vi "Window Maker.vi"(11 "Simple Windows":i32[][](array[numeric])) -> (3 "Plot Bounds":T1[](array[typedef]) {"Plot Bounds (%)"."Bottom (%)" format="%.2f"; "Plot Bounds (%)"."Top (%)" format="%.2f"; "Plot Bounds (%)"."Right (%)" format="%.2f"; "Plot Bounds (%)"."Left (%)" format="%.2f"})   [LabVIEW 2021, in "MultiStokePlot.lvlib" / "MultiPlotPanel.lvclass"]
uses:
  Classes/MultiPlotPanel/MultiPlotPanel.lvclass
  Window Position and plot number.ctl
  Window Position.ctl
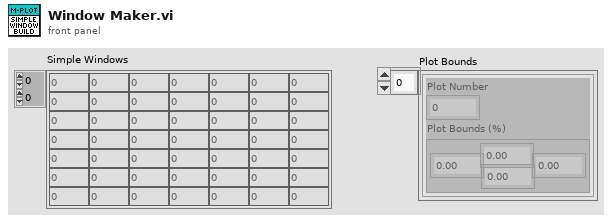
[diagram p1: front panel]
types:
  T1 = typedef "MultiStokePlot.lvlib/MultiPlotPanel.lvclass/Window Position and plot number.ctl" = cluster{"Plot Number":i32, "Plot Bounds (%)":T2}
  T2 = typedef "MultiStokePlot.lvlib/MultiPlotPanel.lvclass/Window Position.ctl" = cluster{"Left (%)":dbl, "Top (%)":dbl, "Right (%)":dbl, "Bottom (%)":dbl}
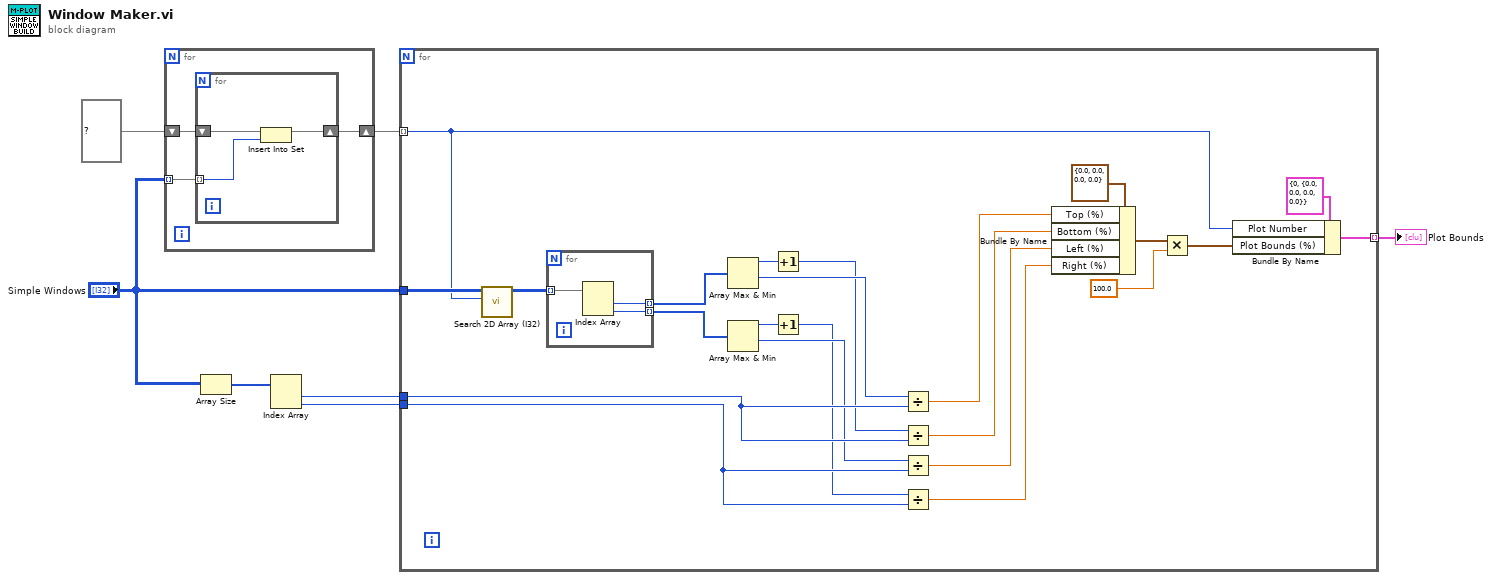
[diagram p0: block diagram]
diagram:
  n1 = for {
    tunnel: "Simple Windows" -> [w10] mode=indexing
    shift-right: [w8] -> w6
    shift-left: set{i32} {} ("set in") -> [w9]
    n2 = for {
      tunnel: w10 -> [w13] mode=indexing
      shift-right: [w11] -> w8
      shift-left: w9 -> [w12]
      n3 = Insert Into Set(10:w13, 11:w12) -> (3:w11:set{i32})  [unwired: 1 out]
    }
  }
  n4 = Array Size(array="Simple Windows") -> (size(s)=w2:i32[])
  n5 = Index Array(array=w2) -> (element #1=w4:i32, element #2=w3:i32)  [unwired: 2 in]
  n6 = for {
    tunnel: "Simple Windows" -> [w36]
    tunnel: w6 -> [w15] mode=indexing
    tunnel: w4 -> [w28]
    tunnel: w3 -> [w31]
    tunnel: [w14] -> w1 mode=indexing
    n7 = call "Search 2D Array (I32).vi"("Element"=w15, "Array"=w36) -> ("Locations"=w35:i32[][])  [unwired: 9 in]
    n8 = for {
      tunnel: w35 -> [w39] mode=indexing
      tunnel: [w38] -> w34 mode=indexing
      tunnel: [w37] -> w33 mode=indexing
      n9 = Index Array(array=w39) -> (element #1=w38:i32, element #2=w37:i32)  [unwired: 2 in]
    }
    n10 = Array Max & Min(array=w34) -> (max value=w25:i32, min value=w27:i32)  [unwired: 2 out]
    n11 = Array Max & Min(array=w33) -> (max value=w23:i32, min value=w26:i32)  [unwired: 2 out]
    n12 = Increment(x=w25) -> (x+1=w24:i32)
    n13 = Increment(x=w23) -> (x+1=w22:i32)
    n14 = Divide(x=w27, y=w28) -> (x/y=w30:dbl)
    n15 = Divide(x=w24, y=w28) -> (x/y=w21:dbl)
    n16 = Divide(x=w26, y=w31) -> (x/y=w29:dbl)
    n17 = Divide(x=w22, y=w31) -> (x/y=w20:dbl)
    n18 = Bundle By Name(cluster=T2 {"Left (%)"=0.0, "Top (%)"=0.0, "Right (%)"=0.0, "Bottom (%)"=0.0} ("Cluster"), "Top (%)"=w30, "Bottom (%)"=w21, "Left (%)"=w29, "Right (%)"=w20) -> (w19:T2)
    n19 = Multiply(x=w19, y=100.0 ("x/y")) -> (x*y=w16:T2)
    n20 = Bundle By Name(cluster=T1 {"Plot Number"=0, "Plot Bounds (%)"={"Left (%)"=0.0, "Top (%)"=0.0, "Right (%)"=0.0, "Bottom (%)"=0.0}} ("Cluster"), "Plot Number"=w15, "Plot Bounds (%)"=w16) -> (w14:T1)
  }
  "Plot Bounds" <- w1
